vi "PicoScope4000GetTimebase2.vi"(4 "Number of Samples":u32, 6 "Memory Segment":u32, 7 "Acquisition Settings":T1 {"postTriggerSamples" format="%_6p"; "preTriggerSamples" format="%_6p"}, 8 "error in (no error)":errorcluster, 9 "oversample":i16, 11 "handle in":i16) -> (0 "error out":errorcluster, 3 "handle out":i16, 5 "Properties Panel":T2 {"Max Total Capture Time Available (sec)" format="%.3p"; "Sample Frequency" format="%.6p"; "Sample Rate" format="%.3p"; "Max Samples Available" format="%_6p"; "Total Capture Time (sec)" format="%.3p"})   [LabVIEW 2009]
doc: "Calls Gettimebase function"
uses:
  ps4000.dll
  shared/Acquisition Settings.ctl
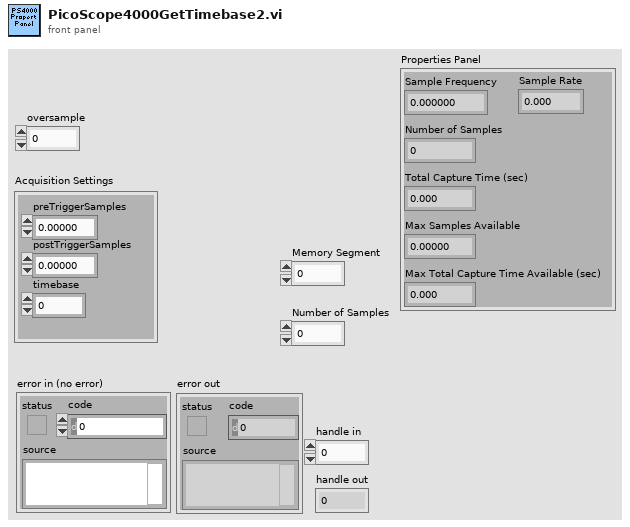
[diagram p1: front panel]
types:
  T1 = typedef "Acquisition Settings.ctl" = cluster{"preTriggerSamples":u64, "postTriggerSamples":u64, "timebase":u32}
  T2 = cluster{"Sample Frequency":dbl, "Sample Rate":dbl, "Max Samples Available":u64, "Number of Samples":u64, "Total Capture Time (sec) ":dbl, "Max Total Capture Time Available (sec)":dbl}
  T3 = cluster{sgl, sgl, "maxSamples":i32, "Number of Samples":u32, sgl, sgl}
  T4 = cluster{dbl, dbl, "maxSamples":i32, "Number of Samples":u32, dbl, dbl}
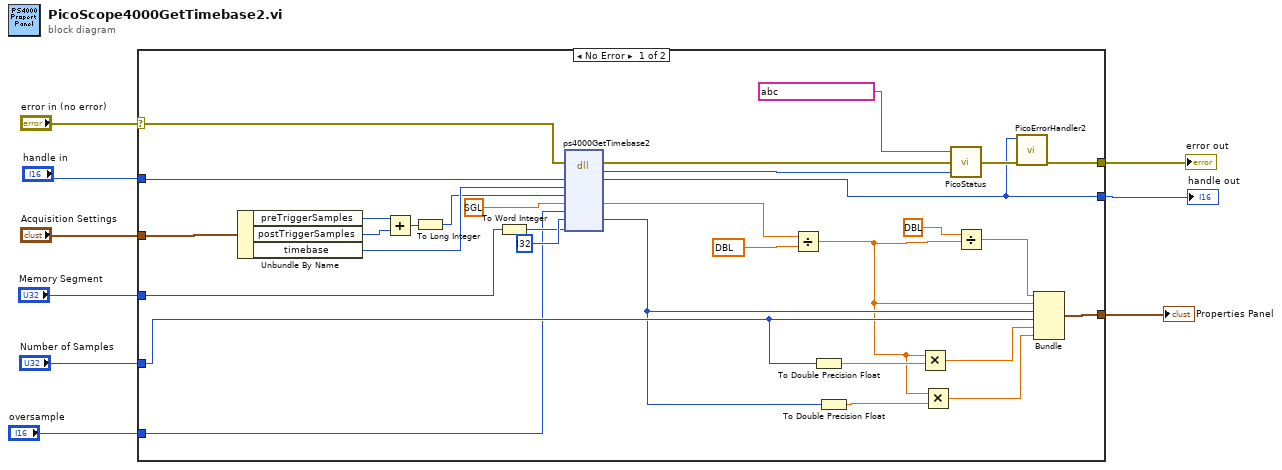
[diagram p0: block diagram]
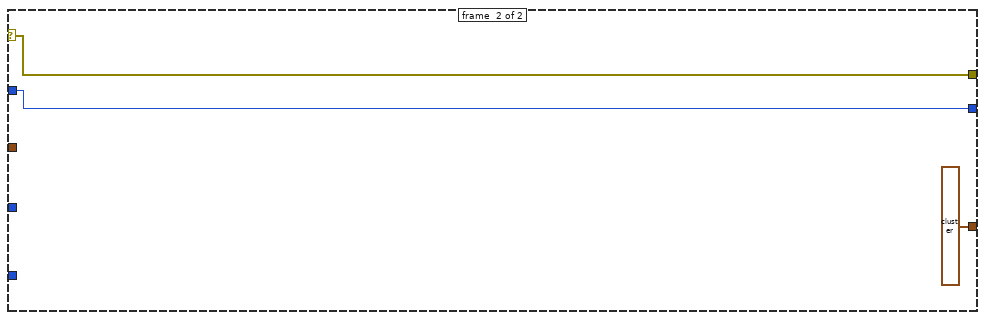
[diagram p2: hidden frame]
diagram:
  n1 = case shown="No Error" "error in (no error)" {
    selector: "error in (no error)" -> [w16 w43]
    tunnel: [w21 w43] -> w9
    tunnel: [w20 w42] -> w8
    tunnel: "Memory Segment" -> [w12 _]
    tunnel: "Number of Samples" -> [w30 _]
    tunnel: "handle in" -> [w15 w42]
    tunnel: [w26 T3 ?] -> w3
    tunnel: "Acquisition Settings" -> [w17 _]
    tunnel: "oversample" -> [w10 _]
    frame #0 {
      n2 = Unbundle By Name(w17) -> ("preTriggerSamples"=w36:u64, "postTriggerSamples"=w37:u64, "timebase"=w38:u32)
      n3 = Add(x=w36, y=w37) -> (x+y=w19:u64)
      n4 = To Long Integer(number=w19) -> (32bit integer=w18:i32)
      n5 = To Word Integer(number=w12) -> (16bit integer=w11:i16)
      n6 = dll-call lib="ps4000.dll" fn="ps4000GetTimebase2"(error in=w16, "handle"=w15, "timebase"=w38, "noSamples"=w18, "timeIntervalNanoseconds"=sgl ?, "oversample"=w10, "maxSamples"=i32 ?, "segmentIndex"=w11) -> (error out=w13:errorcluster, "PICO_STATUS"=w14:u32, "handle"=w20:i16, "timeIntervalNanoseconds"=w39:sgl, "maxSamples"=w28:i32)  [unwired: 6 in, 1 out]
      n7 = Divide(x=w39, y=dbl ?) -> (x/y=w25:dbl)
      n8 = To Double Precision Float(number=w30) -> (double precision float=w32:dbl)
      n9 = To Double Precision Float(number=w28) -> (double precision float=w29:dbl)
      n10 = Multiply(x=w25, y=w32) -> (x*y=w31:dbl)
      n11 = Multiply(x=w25, y=w29) -> (x*y=w27:dbl)
      n12 = call "PicoStatus.vi"("PICO STATUS"=w14, "error in"=w13, "source"=string ?) -> ("error out"=w22:errorcluster)
      n13 = Divide(x=dbl ?, y=w25) -> (x/y=w23:dbl)
      n14 = call "PicoErrorHandler2.vi"("error in (no error)"=w22, "handle In"=w20) -> ("error out"=w21:errorcluster)  [unwired: 9 in]
      n15 = Bundle(w23, w25, "maxSamples"=w28, "Number of Samples"=w30, w31, w27) -> (w26:T4)  [unwired: 1 in]
    }
    frame #1 {
    }
  }
  "error out" <- w9
  "handle out" <- w8
  "Properties Panel" <- w3
